vi "Test_DO.vi"() -> ()   [LabVIEW 2023]
uses:
  DI_DO/DI_DO.lvclass
panel:
  in  "Input":T1
  out "STATUS":string
  out "error out":errorcluster
  out "Error":string
  in  "DO":bool
  in  "PIN":i8
  in  "error in (no error)":errorcluster
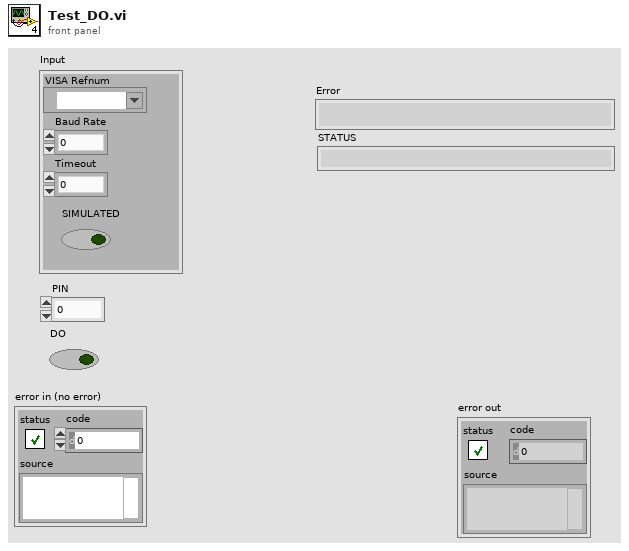
[diagram p1: front panel]
types:
  T1 = cluster{"VISA Refnum":refnum<visa-resource-name>, "Baud Rate":u32, "Timeout":u32, "SIMULATED":bool}
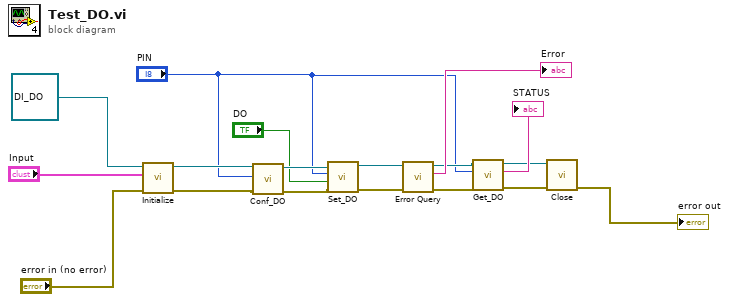
[diagram p0: block diagram]
diagram:
  n1 = call-dynamic "Initialize.vi"("error in (no error)"="error in (no error)", "Input"="Input", "Driver in"=refnum<class "DI_DO.lvclass"> refnum ("Driver_DI_DO.lvlib:DI_DO.lvclass")) -> ("error out"=w17:errorcluster, "Driver out"=w16:refnum<class "DI_DO.lvclass">)  [unwired: 7 in]
  n2 = call-dynamic "Conf_DO.vi"("error in (no error)"=w17, "PIN Number"="PIN", "DI_DO in"=w16) -> ("error out"=w14:errorcluster, "DI_DO out"=w13:refnum<class "DI_DO.lvclass">)  [unwired: 7 in]
  n3 = call-dynamic "Set_DO.vi"("error in (no error)"=w14, "DO"="DO", "PIN"="PIN", "DI_DO in"=w13) -> ("error out"=w11:errorcluster, "DI_DO out"=w10:refnum<class "DI_DO.lvclass">)  [unwired: 6 in]
  n4 = call-dynamic "Error Query.vi"("error in (no error)"=w11, "Driver in"=w10) -> ("error out"=w8:errorcluster, "read buffer"=→"Error":string, "Driver out"=w7:refnum<class "DI_DO.lvclass">)  [unwired: 7 in]
  n5 = call-dynamic "Get_DO.vi"("error in (no error)"=w8, "PIN Number"="PIN", "DI_DO in"=w7) -> ("error out"=w3:errorcluster, "STATUS"=→"STATUS":string, "DI_DO out"=w2:refnum<class "DI_DO.lvclass">)  [unwired: 6 in]
  n6 = call-dynamic "Close.vi"("error in (no error)"=w3, "Driver in"=w2) -> ("error out"=→"error out":errorcluster)  [unwired: 8 in, 1 out]
